vi "tearDown.vi"(8 "error in (no error)":errorcluster, 11 "reference in":refnum<class "Buffers Tests.lvclass">) -> (0 "error out":errorcluster, 3 "reference out":refnum<class "Buffers Tests.lvclass">)   [LabVIEW 2019, in "Buffers Tests.lvclass"]
doc: "tearDown runs after the test method has completed. Use this method to clean up any operations or references that were opened by setUp or the test method. Unit tests should be independent of other unit tests so this VI should ensure that the next test can run in a 'clean' test environment."
uses:
  Buffers Tests.lvclass
  Buffers Tests.lvclass/Buffers Tests.ctl
  Classes/Buffer/Buffer.lvclass
  Classes/Buffers/Buffers.lvclass
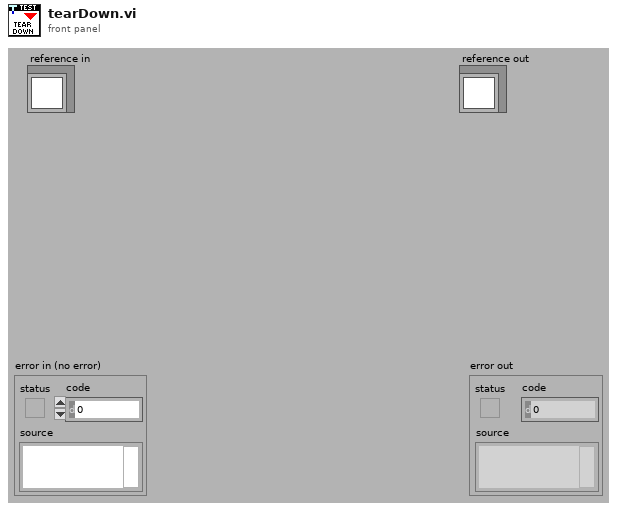
[diagram p1: front panel]
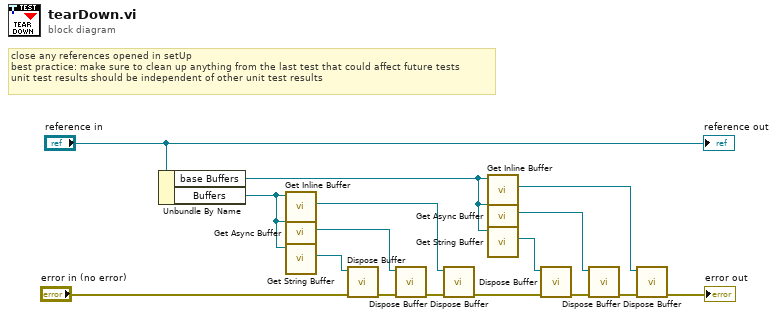
[diagram p0: block diagram]
diagram:
  # "close any references opened in setUp\nbest practice: make sure to clean up anything from the last test that could affect future tests\nunit test results should be independent of other unit test results"
  n1 = Unbundle By Name("reference in") -> ("base Buffers"=w15:refnum<class "Buffers.lvclass">, "Buffers"=w14:refnum<class "Buffers.lvclass">)
  n2 = call "Get Inline Buffer.vi"("Buffers in"=w14) -> ("Inline Buffer"=w7:refnum<class "Buffer.lvclass">)  [unwired: 9 in, 1 out]
  n3 = call "Get Async Buffer.vi"("Buffers in"=w14) -> ("Async Buffer"=w8:refnum<class "Buffer.lvclass">)  [unwired: 9 in, 1 out]
  n4 = call "Get String Buffer.vi"("Buffers in"=w14) -> ("String Buffer"=w9:refnum<class "Buffer.lvclass">)  [unwired: 9 in, 1 out]
  n5 = call "Dispose Buffer.vi"("error in (no error)"="error in (no error)", "Buffer"=w9) -> ("error out"=w11:errorcluster)  [unwired: 8 in, 1 out]
  n6 = call "Dispose Buffer.vi"("error in (no error)"=w11, "Buffer"=w8) -> ("error out"=w10:errorcluster)  [unwired: 8 in, 1 out]
  n7 = call "Dispose Buffer.vi"("error in (no error)"=w10, "Buffer"=w7) -> ("error out"=w6:errorcluster)  [unwired: 8 in, 1 out]
  n8 = call "Get Inline Buffer.vi"("Buffers in"=w15) -> ("Inline Buffer"=w1:refnum<class "Buffer.lvclass">)  [unwired: 9 in, 1 out]
  n9 = call "Get Async Buffer.vi"("Buffers in"=w15) -> ("Async Buffer"=w2:refnum<class "Buffer.lvclass">)  [unwired: 9 in, 1 out]
  n10 = call "Get String Buffer.vi"("Buffers in"=w15) -> ("String Buffer"=w3:refnum<class "Buffer.lvclass">)  [unwired: 9 in, 1 out]
  n11 = call "Dispose Buffer.vi"("error in (no error)"=w6, "Buffer"=w3) -> ("error out"=w5:errorcluster)  [unwired: 8 in, 1 out]
  n12 = call "Dispose Buffer.vi"("error in (no error)"=w5, "Buffer"=w2) -> ("error out"=w4:errorcluster)  [unwired: 8 in, 1 out]
  n13 = call "Dispose Buffer.vi"("error in (no error)"=w4, "Buffer"=w1) -> ("error out"=→"error out":errorcluster)  [unwired: 8 in, 1 out]
  "reference out" <- "reference in"
